vi "VCS Close Device.vi"(8 "error in (no error)":errorcluster, 11 "keyHandle in":u32) -> (0 "error out":errorcluster)   [LabVIEW 2017, in "maxonEPOS.lvlib"]
doc: "<B>VCS Close Device</B> closes the port and releases it for other applications."
uses:
  Examples/maxonEPOS.lvlib
  SSI_Tool/InstrumentsInterfaces/Motordriver/maxon EPOS/Resources/EposCmd.dll
  SSI_Tool/InstrumentsInterfaces/Motordriver/maxon EPOS/Resources/EposCmd64.dll
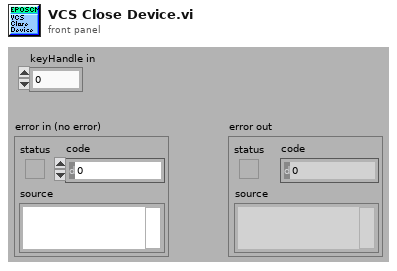
[diagram p1: front panel]
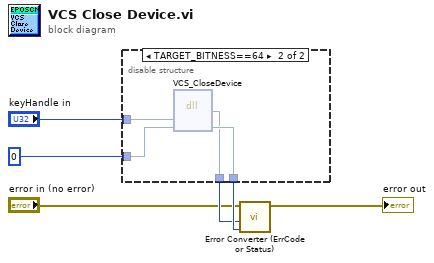
[diagram p0: block diagram]
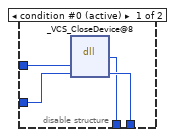
[diagram p2: hidden frame]
diagram:
  n1 = disable-structure shown="TARGET_BITNESS==64" {
    disable-tunnel: u32 0 ("pErrorCode") -> [w10 w14]
    disable-tunnel: [w9 w13] -> w5
    disable-tunnel: [w8 w12] -> w4
    disable-tunnel: "keyHandle in" -> [w7 w11]
    frame condition #0 (active) {
      n2 = dll-call lib="C:/workspace/project/scancon/sw/SSI_Tool/InstrumentsInterfaces/Motordriver/maxon EPOS/Resources/EposCmd.*" fn="_VCS_CloseDevice@8"("KeyHandle"=w7, "pErrorCode"=w10) -> ("return type"=w8:i32, "pErrorCode"=w9:u32)  [unwired: 4 in, 2 out]
    }
    frame condition #1 {
      n3 = dll-call lib="C:/LabVIEW/maxon EPOS/Resources/EposCmd64.dll" fn="VCS_CloseDevice" ("EposCmd.dll:_VCS_CloseDevice@8")("KeyHandle"=w11, "pErrorCode"=w14) -> ("return type"=w12:i32, "pErrorCode"=w13:u32)  [unwired: 4 in, 2 out]
    }
  }
  n4 = call "Error Converter (ErrCode or Status).vi"("error code"=w5, "return type"=w4, "error in (no error)"="error in (no error)") -> ("error out"=→"error out":errorcluster)  [unwired: 7 in]
